vi "TAT-Main.vi"() -> ()   [LabVIEW 2017]
panel:
  in  "Modify SN":bool
  in  "PRINT":bool
  in  "Torque IO Status":bool
  in  "Ass IO Status":bool
  in  "Recipe":bool
  out "error out":errorcluster
  in  "Logout":bool
  in  "Stop":bool
  in  "Create Login":bool
  in  "Reports":bool
  in  "Start":bool
  out "Time":string
  out "Date":string
  in  "Login":bool
  # "STRUT PERIFERAL ASS. MACHINE"
  # "Contact:-- +91 9325640282"
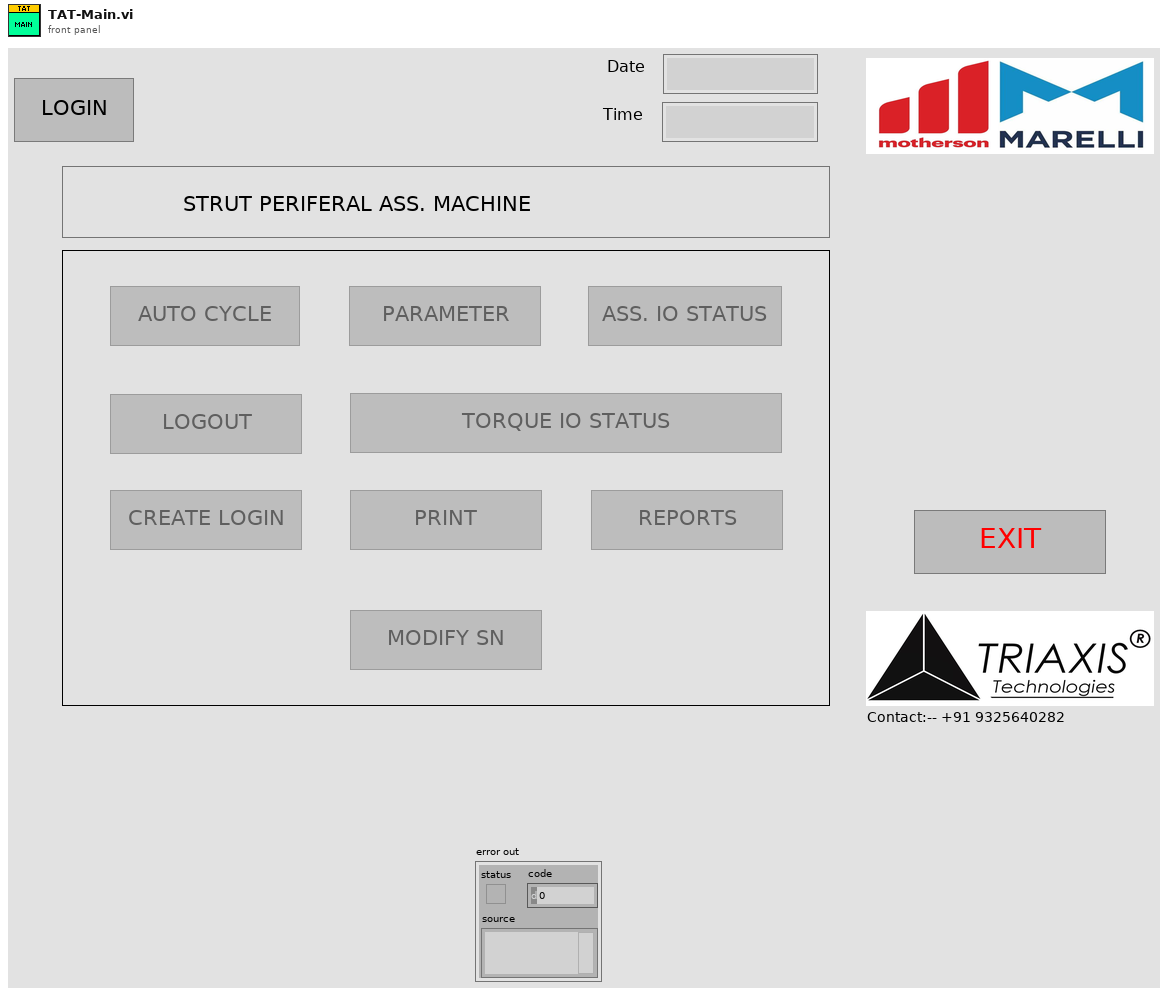
[diagram p1: front panel]
types:
  T1 = enum8{"Enabled", "Disabled", "Disabled and Grayed Out"}
  T2 = enum32{"Invalid", "Standard", "Closed", "Hidden", "Minimized", "Maximized"}
  T3 = enum32{"invalid app kind", "Development System", "Run Time System", "Student Edition", "Embedded LabVIEW", "Evaluation", "Custom"}
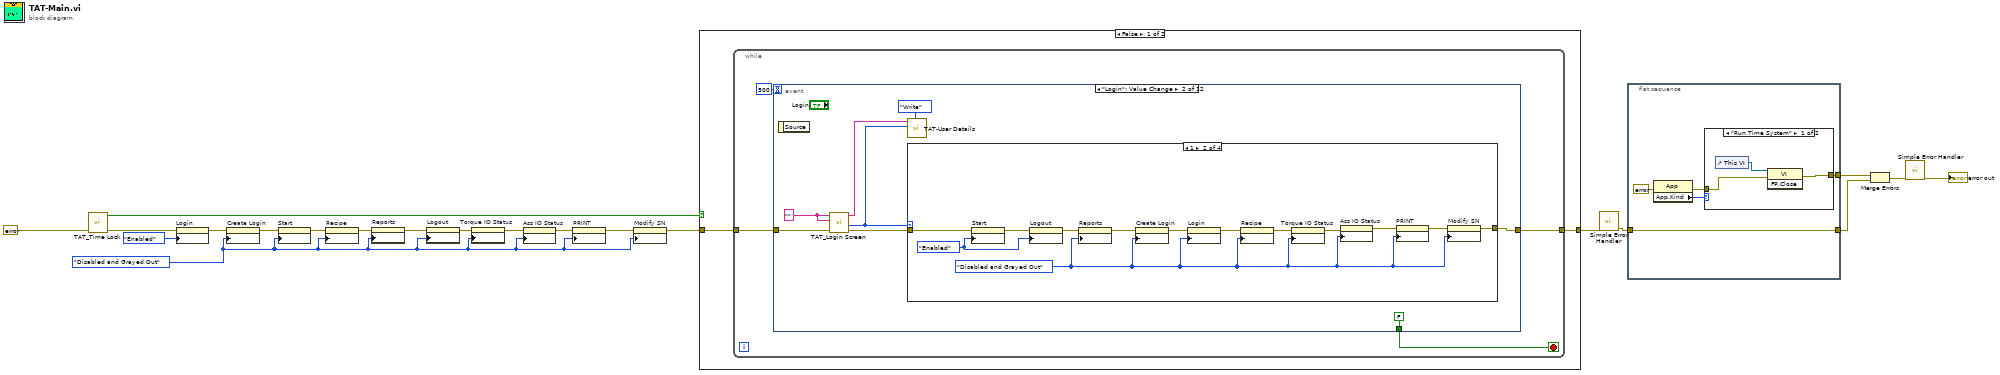
[diagram p0: block diagram]
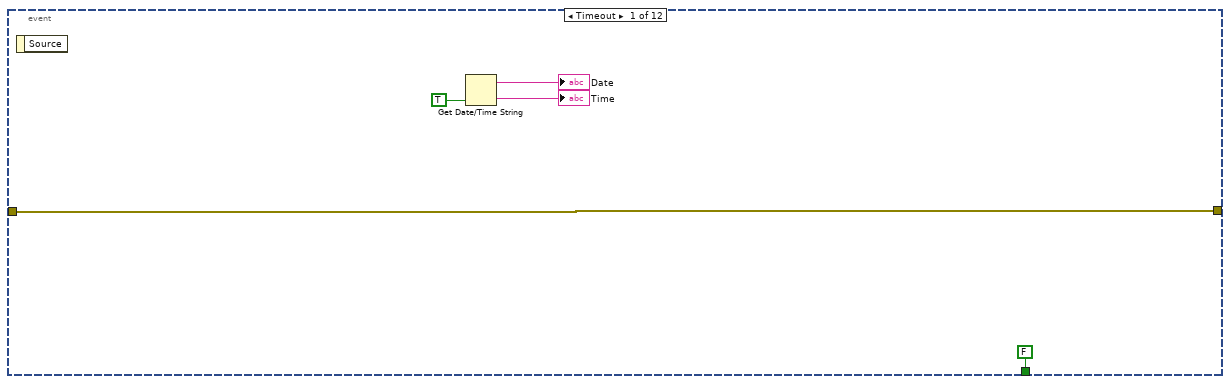
[diagram p3: hidden frame]
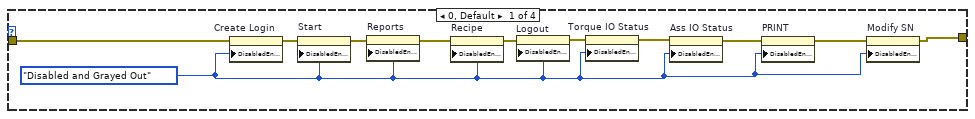
[diagram p4: hidden frame]
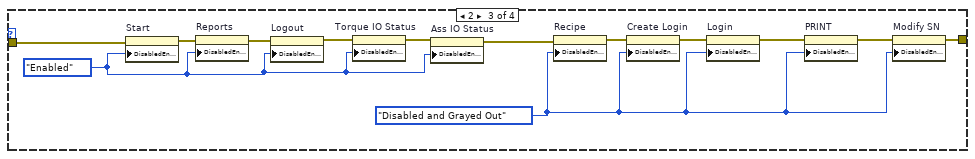
[diagram p5: hidden frame]
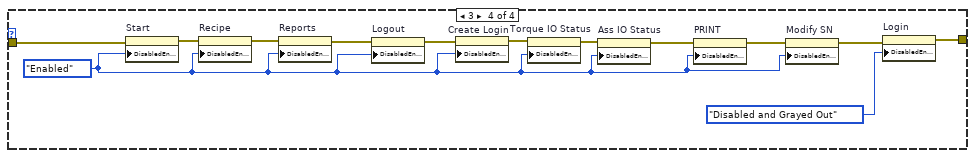
[diagram p6: hidden frame]
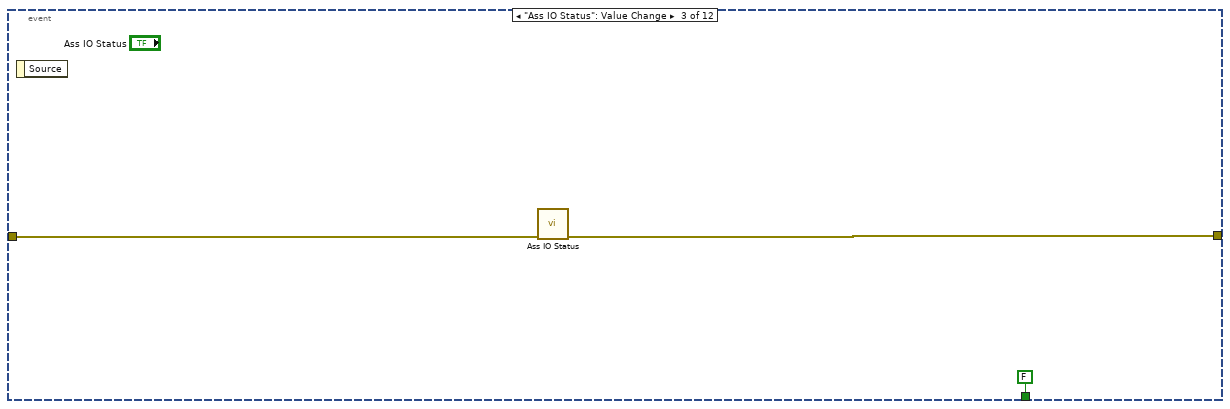
[diagram p7: hidden frame]
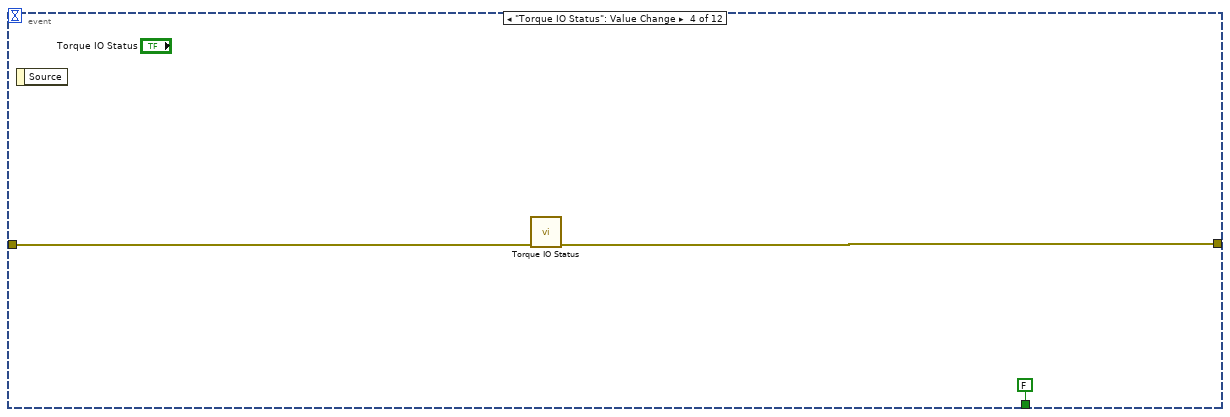
[diagram p8: hidden frame]
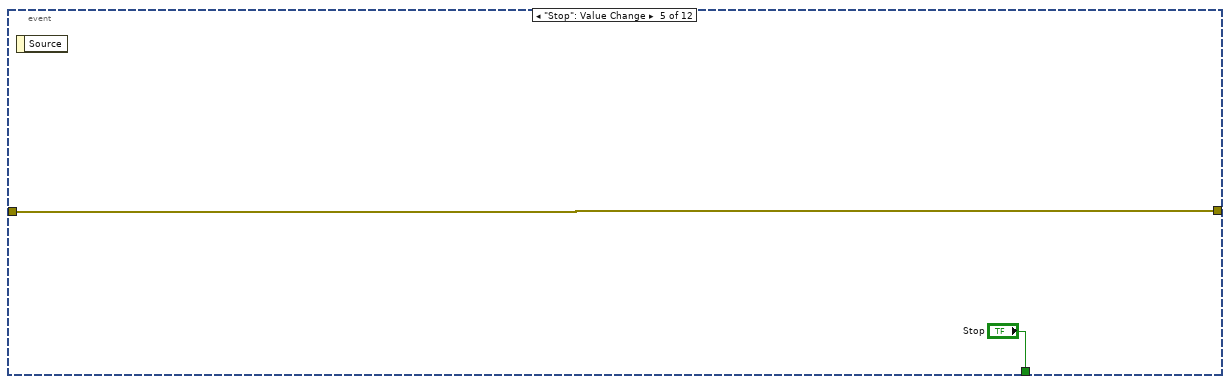
[diagram p9: hidden frame]
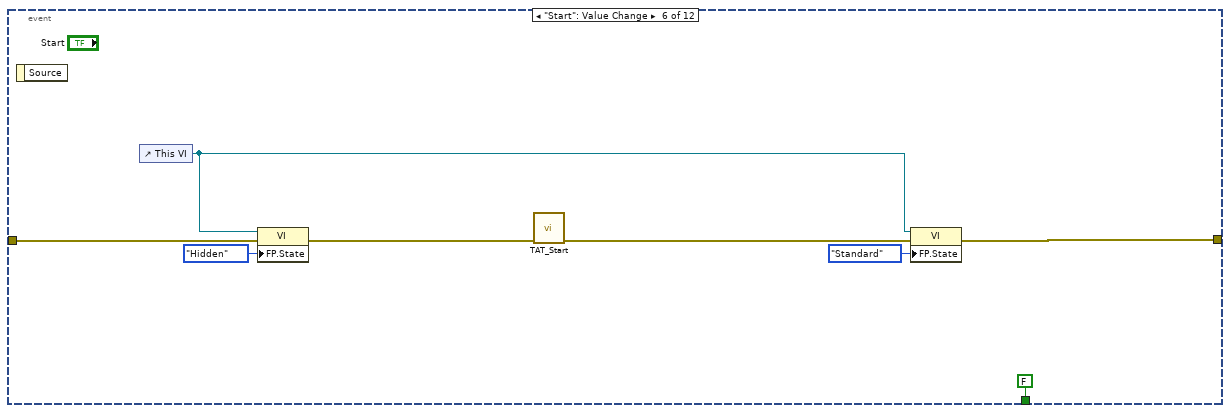
[diagram p10: hidden frame]
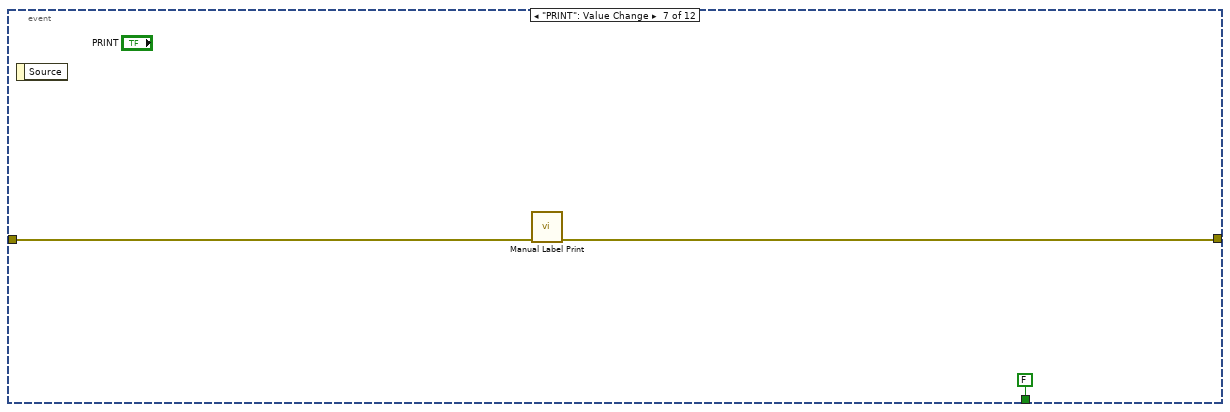
[diagram p11: hidden frame]
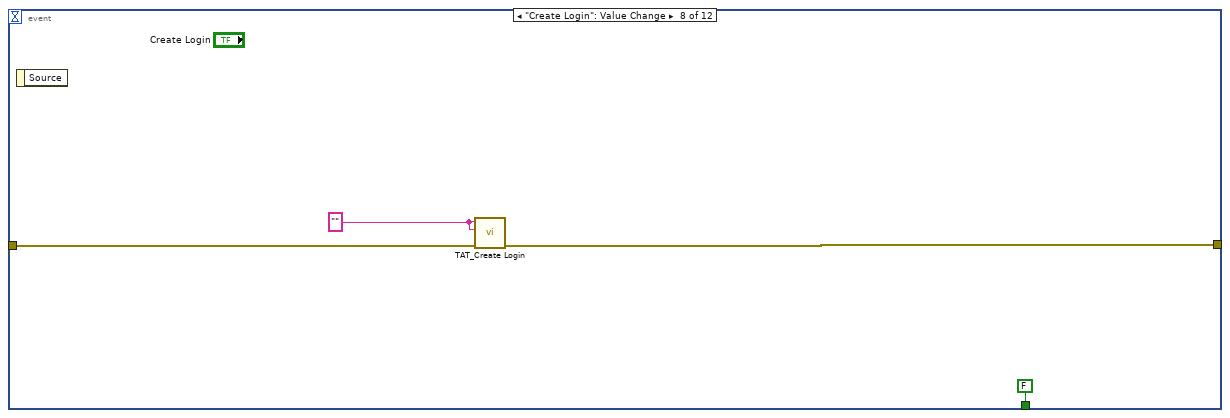
[diagram p12: hidden frame]
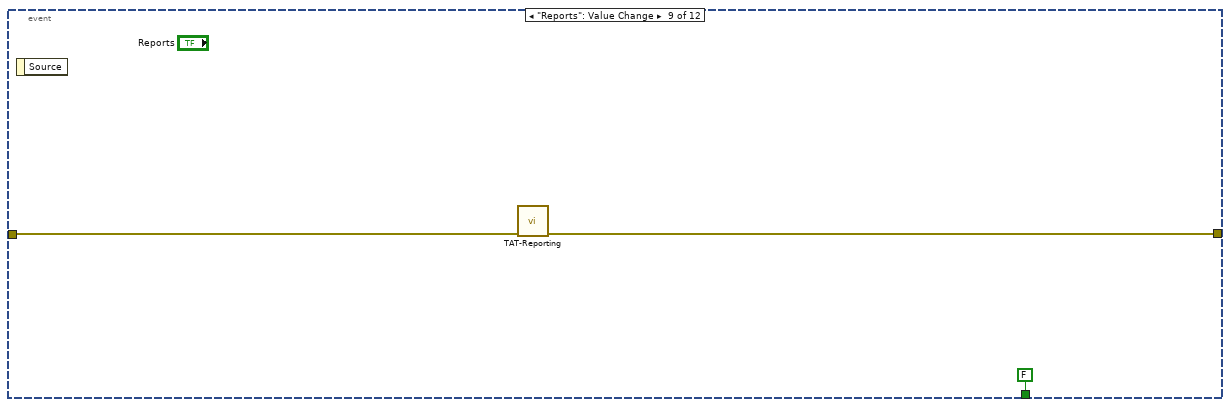
[diagram p13: hidden frame]
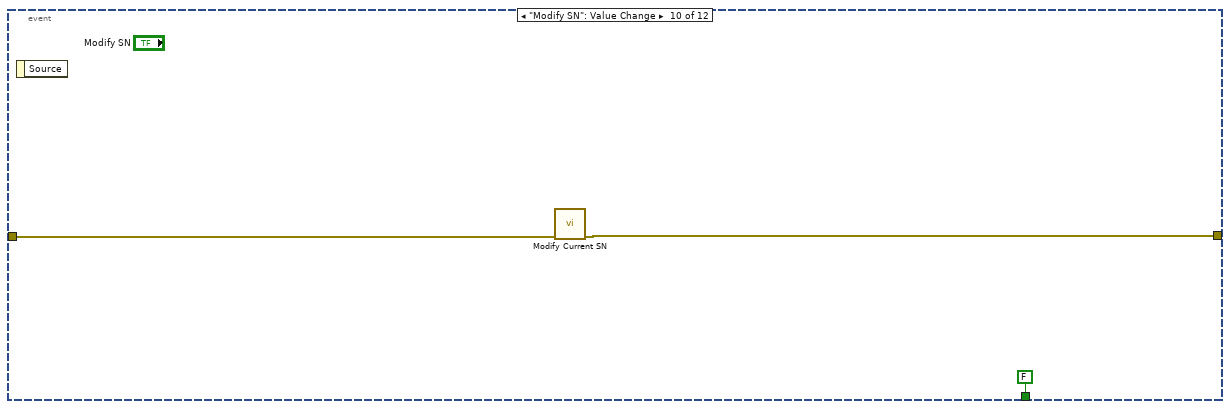
[diagram p14: hidden frame]
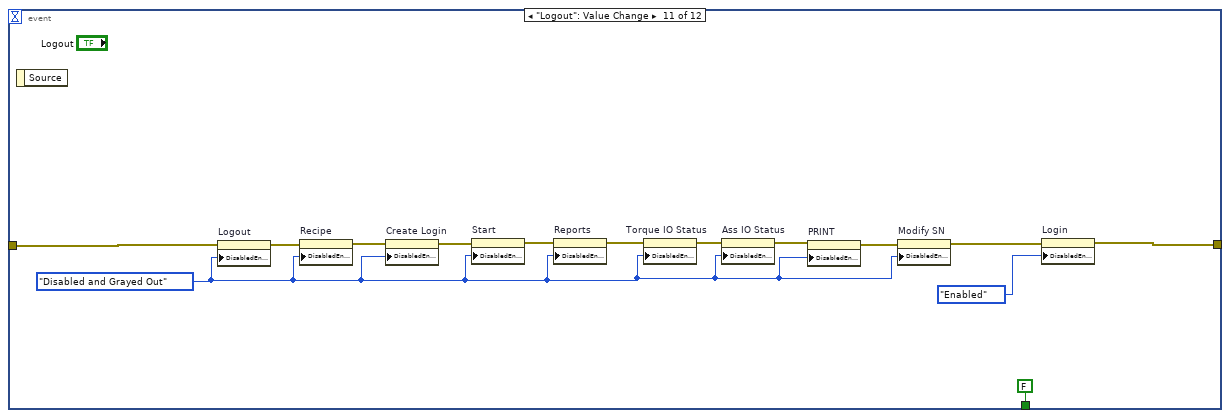
[diagram p15: hidden frame]
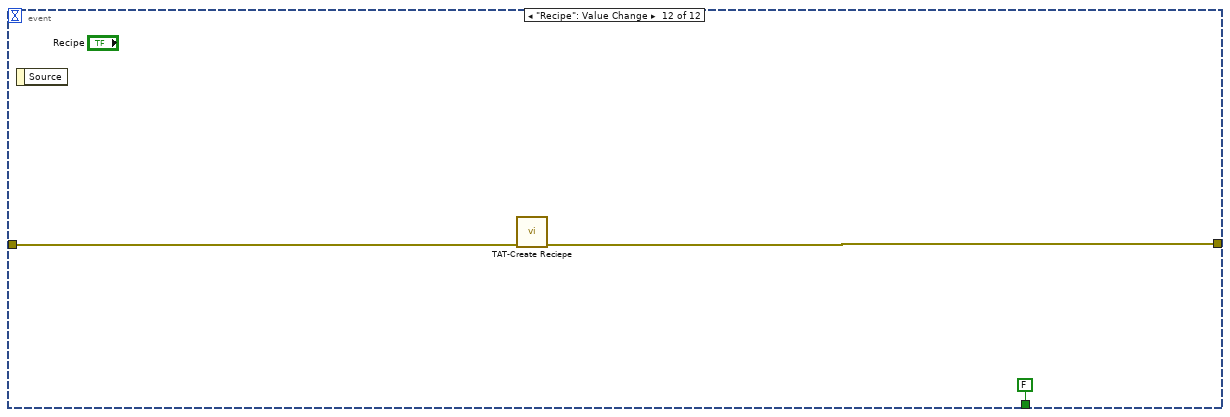
[diagram p16: hidden frame]
diagram:
  w1 = T1."Disabled and Grayed Out" ("Disabled")
  n1 = call "TAT_Time Lock.vi"("error in"=errorcluster {"status"=FALSE, "code"=0, "source"=""} ("error constant")) -> ("error out"=w13:errorcluster, "Time Laps or MAC ?"=w20:bool)  [unwired: 9 in]
  n2 = property on="Login" class="Bool"(error in=w13, "DisabledEnum"=T1."Enabled" ("Disabled")) -> (error out=w12:errorcluster)  [unwired: 1 in, 1 out]
  n3 = property on="Create Login" class="Bool"(error in=w12, "DisabledEnum"=w1) -> (error out=w18:errorcluster)  [unwired: 1 in, 1 out]
  n4 = property on="Start" class="Bool"(error in=w18, "DisabledEnum"=w1) -> (error out=w8:errorcluster)  [unwired: 1 in, 1 out]
  n5 = property on="Recipe" class="Bool"(error in=w8, "DisabledEnum"=w1) -> (error out=w7:errorcluster)  [unwired: 1 in, 1 out]
  n6 = property on="Reports" class="Bool"(error in=w7, "DisabledEnum"=w1) -> (error out=w10:errorcluster)  [unwired: 1 in, 1 out]
  n7 = property on="Logout" class="Bool"(error in=w10, "DisabledEnum"=w1) -> (error out=w6:errorcluster)  [unwired: 1 in, 1 out]
  n8 = property on="Torque IO Status" class="Bool"(error in=w6, "DisabledEnum"=w1) -> (error out=w5:errorcluster)  [unwired: 1 in, 1 out]
  n9 = property on="Ass IO Status" class="Bool"(error in=w5, "DisabledEnum"=w1) -> (error out=w4:errorcluster)  [unwired: 1 in, 1 out]
  n10 = property on="PRINT" class="Bool"(error in=w4, "DisabledEnum"=w1) -> (error out=w3:errorcluster)  [unwired: 1 in, 1 out]
  n11 = property on="Modify SN" class="Bool"(error in=w3, "DisabledEnum"=w1) -> (error out=w2:errorcluster)  [unwired: 1 in, 1 out]
  n12 = case shown="False" w20 {
    tunnel: w2 -> [w23 w137]
    tunnel: [w22 w137] -> w19
    frame False {
      n13 = while {
        tunnel: w23 -> [w26]
        tunnel: [w25] -> w22
        stop <- w24 stop-if-true
        n14 = event shown="[1] \"Login\": Value Change" {
          selector: _ -> [_ _ _ _ _ _ _ _ _ _ _ _]
          dyn-events: _ -> [_ _ _ _ _ _ _ _ _ _ _ _]
          timeout: 500 -> [_ _ _ _ _ _ _ _ _ _ _ _]
          tunnel: w26 -> [w30 w40 w93 w95 w97 w104 w108 w113 w116 w119 w130 w136]
          tunnel: [w30 w38 w92 w94 w97 w101 w107 w112 w115 w118 w131 w135] -> w25
          tunnel: [FALSE ("Stop") FALSE ("Stop") FALSE ("Stop") FALSE ("Stop") "Stop" FALSE ("Stop") FALSE ("Stop") FALSE ("Stop") FALSE ("Stop") FALSE ("Stop") FALSE ("Stop") FALSE ("Stop")] -> w24
          event Timeout {
            n15 = event-data() -> ()  [unwired: 1 in, 1 out]
            n16 = Get Date/Time String(want seconds? (F)=TRUE) -> (date string=→"Date":string, time string=→"Time":string)  [unwired: 2 in]
          }
          event "Login": Value Change {
            w35 = "" ("User Name")
            n17 = event-data() -> ()  [unwired: 1 in, 1 out]
            n18 = call "TAT_Login Screen.vi"("Error In"=w40, "Password"=w35, "User Name"=w35) -> ("error out"=w39:errorcluster, "Level"=w33:i32, "User Name Out"=w36:string)  [unwired: 5 in, 1 out]
            n19 = call "TAT-User Details.vi"("Enum"=enum16{"Read", "Write"}."Write", "Level In"=w33, "User Name In"=w36) -> ()  [unwired: 7 in, 2 out]
            n20 = case shown="1" w33 {
              tunnel: w39 -> [w49 w64 w77 w90]
              tunnel: [w42 w53 w66 w89] -> w38
              frame 0, Default {
                w41 = T1."Disabled and Grayed Out" ("Disabled")
                n21 = property on="Create Login" class="Bool"(error in=w49, "DisabledEnum"=w41) -> (error out=w51:errorcluster)  [unwired: 1 in, 1 out]
                n22 = property on="Start" class="Bool"(error in=w51, "DisabledEnum"=w41) -> (error out=w50:errorcluster)  [unwired: 1 in, 1 out]
                n23 = property on="Reports" class="Bool"(error in=w50, "DisabledEnum"=w41) -> (error out=w48:errorcluster)  [unwired: 1 in, 1 out]
                n24 = property on="Recipe" class="Bool"(error in=w48, "DisabledEnum"=w41) -> (error out=w47:errorcluster)  [unwired: 1 in, 1 out]
                n25 = property on="Logout" class="Bool"(error in=w47, "DisabledEnum"=w41) -> (error out=w46:errorcluster)  [unwired: 1 in, 1 out]
                n26 = property on="Torque IO Status" class="Bool"(error in=w46, "DisabledEnum"=w41) -> (error out=w45:errorcluster)  [unwired: 1 in, 1 out]
                n27 = property on="Ass IO Status" class="Bool"(error in=w45, "DisabledEnum"=w41) -> (error out=w44:errorcluster)  [unwired: 1 in, 1 out]
                n28 = property on="PRINT" class="Bool"(error in=w44, "DisabledEnum"=w41) -> (error out=w43:errorcluster)  [unwired: 1 in, 1 out]
                n29 = property on="Modify SN" class="Bool"(error in=w43, "DisabledEnum"=w41) -> (error out=w42:errorcluster)  [unwired: 1 in, 1 out]
              }
              frame 1 {
                w52 = T1."Disabled and Grayed Out" ("Disabled")
                w60 = T1."Enabled" ("Disabled")
                n30 = property on="Start" class="Bool"(error in=w64, "DisabledEnum"=w60) -> (error out=w59:errorcluster)  [unwired: 1 in, 1 out]
                n31 = property on="Logout" class="Bool"(error in=w59, "DisabledEnum"=w60) -> (error out=w62:errorcluster)  [unwired: 1 in, 1 out]
                n32 = property on="Reports" class="Bool"(error in=w62, "DisabledEnum"=w52) -> (error out=w63:errorcluster)  [unwired: 1 in, 1 out]
                n33 = property on="Create Login" class="Bool"(error in=w63, "DisabledEnum"=w52) -> (error out=w61:errorcluster)  [unwired: 1 in, 1 out]
                n34 = property on="Login" class="Bool"(error in=w61, "DisabledEnum"=w52) -> (error out=w58:errorcluster)  [unwired: 1 in, 1 out]
                n35 = property on="Recipe" class="Bool"(error in=w58, "DisabledEnum"=w52) -> (error out=w56:errorcluster)  [unwired: 1 in, 1 out]
                n36 = property on="Torque IO Status" class="Bool"(error in=w56, "DisabledEnum"=w52) -> (error out=w57:errorcluster)  [unwired: 1 in, 1 out]
                n37 = property on="Ass IO Status" class="Bool"(error in=w57, "DisabledEnum"=w52) -> (error out=w55:errorcluster)  [unwired: 1 in, 1 out]
                n38 = property on="PRINT" class="Bool"(error in=w55, "DisabledEnum"=w52) -> (error out=w54:errorcluster)  [unwired: 1 in, 1 out]
                n39 = property on="Modify SN" class="Bool"(error in=w54, "DisabledEnum"=w52) -> (error out=w53:errorcluster)  [unwired: 1 in, 1 out]
              }
              frame 2 {
                w65 = T1."Disabled and Grayed Out" ("Disabled")
                w69 = T1."Enabled" ("Disabled")
                n40 = property on="Start" class="Bool"(error in=w77, "DisabledEnum"=w69) -> (error out=w74:errorcluster)  [unwired: 1 in, 1 out]
                n41 = property on="Reports" class="Bool"(error in=w74, "DisabledEnum"=w69) -> (error out=w76:errorcluster)  [unwired: 1 in, 1 out]
                n42 = property on="Logout" class="Bool"(error in=w76, "DisabledEnum"=w69) -> (error out=w71:errorcluster)  [unwired: 1 in, 1 out]
                n43 = property on="Torque IO Status" class="Bool"(error in=w71, "DisabledEnum"=w69) -> (error out=w72:errorcluster)  [unwired: 1 in, 1 out]
                n44 = property on="Ass IO Status" class="Bool"(error in=w72, "DisabledEnum"=w69) -> (error out=w70:errorcluster)  [unwired: 1 in, 1 out]
                n45 = property on="Recipe" class="Bool"(error in=w70, "DisabledEnum"=w65) -> (error out=w73:errorcluster)  [unwired: 1 in, 1 out]
                n46 = property on="Create Login" class="Bool"(error in=w73, "DisabledEnum"=w65) -> (error out=w75:errorcluster)  [unwired: 1 in, 1 out]
                n47 = property on="Login" class="Bool"(error in=w75, "DisabledEnum"=w65) -> (error out=w68:errorcluster)  [unwired: 1 in, 1 out]
                n48 = property on="PRINT" class="Bool"(error in=w68, "DisabledEnum"=w65) -> (error out=w67:errorcluster)  [unwired: 1 in, 1 out]
                n49 = property on="Modify SN" class="Bool"(error in=w67, "DisabledEnum"=w65) -> (error out=w66:errorcluster)  [unwired: 1 in, 1 out]
              }
              frame 3 {
                w78 = T1."Enabled" ("Disabled")
                n50 = property on="Start" class="Bool"(error in=w90, "DisabledEnum"=w78) -> (error out=w85:errorcluster)  [unwired: 1 in, 1 out]
                n51 = property on="Recipe" class="Bool"(error in=w85, "DisabledEnum"=w78) -> (error out=w84:errorcluster)  [unwired: 1 in, 1 out]
                n52 = property on="Reports" class="Bool"(error in=w84, "DisabledEnum"=w78) -> (error out=w87:errorcluster)  [unwired: 1 in, 1 out]
                n53 = property on="Logout" class="Bool"(error in=w87, "DisabledEnum"=w78) -> (error out=w86:errorcluster)  [unwired: 1 in, 1 out]
                n54 = property on="Create Login" class="Bool"(error in=w86, "DisabledEnum"=w78) -> (error out=w83:errorcluster)  [unwired: 1 in, 1 out]
                n55 = property on="Torque IO Status" class="Bool"(error in=w83, "DisabledEnum"=w78) -> (error out=w82:errorcluster)  [unwired: 1 in, 1 out]
                n56 = property on="Ass IO Status" class="Bool"(error in=w82, "DisabledEnum"=w78) -> (error out=w81:errorcluster)  [unwired: 1 in, 1 out]
                n57 = property on="PRINT" class="Bool"(error in=w81, "DisabledEnum"=w78) -> (error out=w80:errorcluster)  [unwired: 1 in, 1 out]
                n58 = property on="Modify SN" class="Bool"(error in=w80, "DisabledEnum"=w78) -> (error out=w79:errorcluster)  [unwired: 1 in, 1 out]
                n59 = property on="Login" class="Bool"(error in=w79, "DisabledEnum"=T1."Disabled and Grayed Out" ("Disabled")) -> (error out=w89:errorcluster)  [unwired: 1 in, 1 out]
              }
            }
          }
          event "Ass IO Status": Value Change {
            n60 = event-data() -> ()  [unwired: 1 in, 1 out]
            n61 = call "Ass IO Status.vi"("error in (no error)"=w93) -> ("error out"=w92:errorcluster)  [unwired: 10 in]
          }
          event "Torque IO Status": Value Change {
            n62 = event-data() -> ()  [unwired: 1 in, 1 out]
            n63 = call "Torque IO Status.vi"("error in (no error)"=w95) -> ("error out"=w94:errorcluster)  [unwired: 10 in]
          }
          event "Stop": Value Change {
            n64 = event-data() -> ()  [unwired: 1 in, 1 out]
          }
          event "Start": Value Change {
            n65 = event-data() -> ()  [unwired: 1 in, 1 out]
            n66 = control-ref of="This VI"() -> (w102:refnum<vi>)
            n67 = property class="VI"(reference=w102, error in=w104, "FP.State"=T2."Hidden" ("Front Panel Window:State")) -> (error out=w100:errorcluster)  [unwired: 1 out]
            n68 = call "TAT_Start.vi"("error In"=w100) -> ("error Out"=w99:errorcluster)  [unwired: 10 in]
            n69 = property class="VI"(reference=w102, error in=w99, "FP.State"=T2."Standard" ("Front Panel Window:State")) -> (error out=w101:errorcluster)  [unwired: 1 out]
          }
          event "PRINT": Value Change {
            n70 = event-data() -> ()  [unwired: 1 in, 1 out]
            n71 = call "Manual Label Print.vi"("error in (no error)"=w108) -> ("error out"=w107:errorcluster)  [unwired: 10 in]
          }
          event "Create Login": Value Change {
            w111 = "" ("User Name")
            n72 = event-data() -> ()  [unwired: 1 in, 1 out]
            n73 = call "TAT_Create Login.vi"("Error In"=w113, "Password"=w111, "User Name"=w111) -> ("error out"=w112:errorcluster)  [unwired: 6 in]
          }
          event "Reports": Value Change {
            n74 = event-data() -> ()  [unwired: 1 in, 1 out]
            n75 = call "TAT-Reporting.vi"("error in (no error)"=w116) -> ("error out"=w115:errorcluster)  [unwired: 10 in]
          }
          event "Modify SN": Value Change {
            n76 = event-data() -> ()  [unwired: 1 in, 1 out]
            n77 = call "Modify Current SN.vi"("error in (no error)"=w119) -> ("error out"=w118:errorcluster)  [unwired: 10 in]
          }
          event "Logout": Value Change {
            w120 = T1."Disabled and Grayed Out" ("Disabled")
            n78 = event-data() -> ()  [unwired: 1 in, 1 out]
            n79 = property on="Logout" class="Bool"(error in=w130, "DisabledEnum"=w120) -> (error out=w128:errorcluster)  [unwired: 1 in, 1 out]
            n80 = property on="Recipe" class="Bool"(error in=w128, "DisabledEnum"=w120) -> (error out=w127:errorcluster)  [unwired: 1 in, 1 out]
            n81 = property on="Create Login" class="Bool"(error in=w127, "DisabledEnum"=w120) -> (error out=w133:errorcluster)  [unwired: 1 in, 1 out]
            n82 = property on="Start" class="Bool"(error in=w133, "DisabledEnum"=w120) -> (error out=w132:errorcluster)  [unwired: 1 in, 1 out]
            n83 = property on="Reports" class="Bool"(error in=w132, "DisabledEnum"=w120) -> (error out=w125:errorcluster)  [unwired: 1 in, 1 out]
            n84 = property on="Torque IO Status" class="Bool"(error in=w125, "DisabledEnum"=w120) -> (error out=w126:errorcluster)  [unwired: 1 in, 1 out]
            n85 = property on="Ass IO Status" class="Bool"(error in=w126, "DisabledEnum"=w120) -> (error out=w123:errorcluster)  [unwired: 1 in, 1 out]
            n86 = property on="PRINT" class="Bool"(error in=w123, "DisabledEnum"=w120) -> (error out=w122:errorcluster)  [unwired: 1 in, 1 out]
            n87 = property on="Modify SN" class="Bool"(error in=w122, "DisabledEnum"=w120) -> (error out=w121:errorcluster)  [unwired: 1 in, 1 out]
            n88 = property on="Login" class="Bool"(error in=w121, "DisabledEnum"=T1."Enabled" ("Disabled")) -> (error out=w131:errorcluster)  [unwired: 1 in, 1 out]
          }
          event "Recipe": Value Change {
            n89 = event-data() -> ()  [unwired: 1 in, 1 out]
            n90 = call "TAT-Create Reciepe.vi"("Error In"=w136) -> ("error out"=w135:errorcluster)  [unwired: 10 in]
          }
        }
      }
    }
    frame True {
    }
  }
  n91 = call <vilib>:"Simple Error Handler.vi"("error in (no error)"=w19) -> ("error out"=w14:errorcluster)  [unwired: 4 in, 4 out]
  n92 = flat-sequence {
    tunnel: [w139] -> w17
    tunnel: [w138] -> w15
    tunnel: w14 -> [w138]
    frame #0 {
      n93 = property class="App"(error in=errorcluster {"status"=FALSE, "code"=0, "source"=""} ("error in (no error)")) -> (error out=w141:errorcluster, "App.Kind"=w142:T3)  [unwired: 1 in, 1 out]
      n94 = case shown="\"Run Time System\"" w142 {
        tunnel: w141 -> [w144 w146]
        tunnel: [w143 w146] -> w139
        frame "Run Time System" {
          n95 = control-ref of="This VI"() -> (w145:refnum<vi>)
          n96 = invoke class="VI" method="FP.Close"(reference=w145, error in=w144) -> (error out=w143:errorcluster)  [unwired: 1 in, 2 out]
        }
        frame "Development System", Default {
        }
      }
    }
  }
  n97 = Merge Errors(w17, w15) -> (w16:errorcluster)
  n98 = call <vilib>:"Simple Error Handler.vi"("error in (no error)"=w16) -> ("error out"=→"error out":errorcluster)  [unwired: 4 in, 4 out]
